vi "Initialize.vi"(8 "error in (no error)":errorcluster, 11 "Camera_Prime95B in":refnum<class "Camera_Prime95B.lvclass">) -> (0 "error out":errorcluster, 3 "Camera_Prime95B out":refnum<class "Camera_Prime95B.lvclass">)   [LabVIEW 2020, in "Camera_Prime95B.lvlib" / "Camera_Prime95B.lvclass"]
uses:
  Camera_Prime95B.lvclass
  E:/Development/DevHardSoftware/MicroscopyFramework/Model/Hardware Layer/Real Hardware/Camera_Prime95B/Camera_Prime95B/Dependencies/PVCamNET.dll
  Dependencies/PVCamNET.dll
  Hardware Abstraction Layer/Component/Camera/Camera/Camera.lvclass
  Hardware Abstraction Layer/Component/Device/Device/DeviceStatus.ctl
  Hardware Abstraction Layer/Component/Device/Device/Device.lvlib
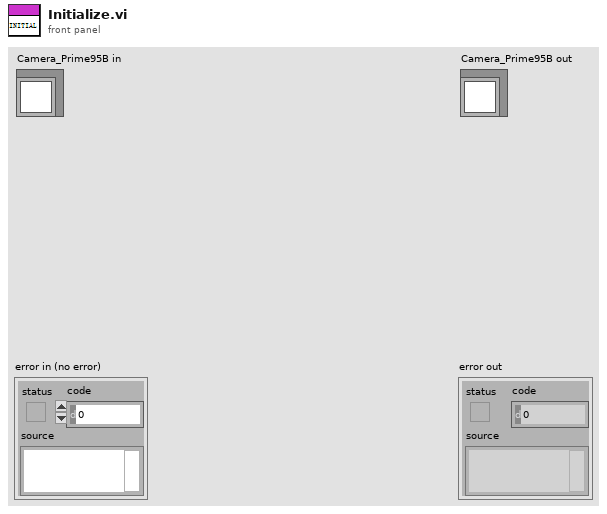
[diagram p1: front panel]
types:
  T1 = typedef "Device.lvlib/DeviceStatus.ctl" = i32
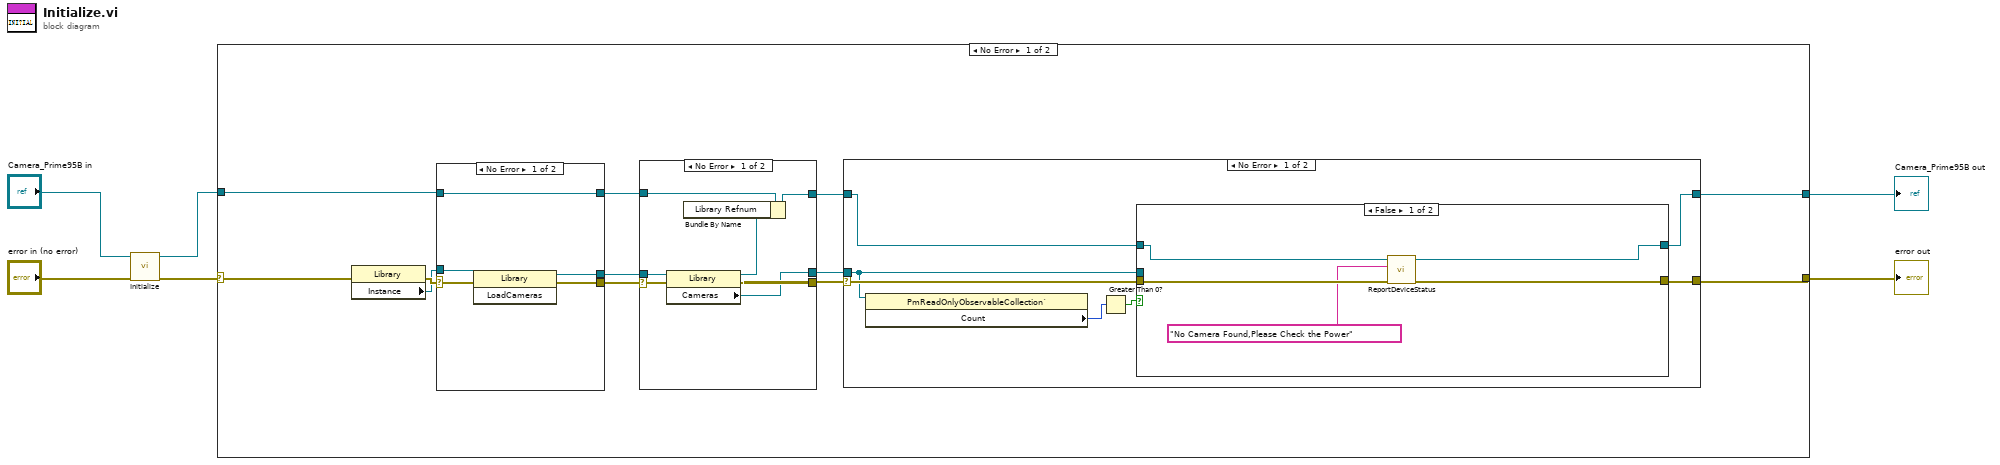
[diagram p0: block diagram]
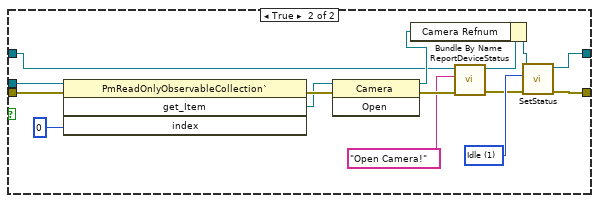
[diagram p2: hidden frame]
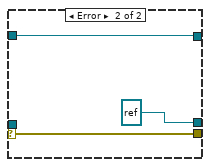
[diagram p4: hidden frame]
diagram:
  n1 = call-parent "Initialize.vi"("error in (no error)"="error in (no error)", "Camera in"="Camera_Prime95B in") -> ("error out"=w2:errorcluster, "Camera out"=w1:refnum<class "Camera_Prime95B.lvclass">)  [unwired: 8 in]
  n2 = case shown="No Error" w2 {
    selector: w2 -> [w12 w67]
    tunnel: [w8 w67] -> w5
    tunnel: w1 -> [w11 w66]
    tunnel: [w7 w66] -> w6
    frame No Error {
      n3 = property class="Library"(error in=w12) -> (error out=w18:errorcluster, "Instance"=w15:refnum<k24>)  [unwired: 1 in, 1 out]
      n4 = case shown="No Error" w18 {
        selector: w18 -> [w60 w65]
        tunnel: [w61 w65] -> w16
        tunnel: [w62 w64] -> w17
        tunnel: w15 -> [w59 w64]
        tunnel: w11 -> [w58 w63]
        tunnel: [w58 w63] -> w10
        frame No Error {
          n5 = invoke class="Library" method="LoadCameras"(reference=w59, error in=w60) -> (reference out=w62:refnum<k24>, error out=w61:errorcluster)  [unwired: 1 in, 1 out]
        }
        frame Error {
        }
      }
      n6 = case shown="No Error" w16 {
        selector: w16 -> [w54 w57]
        tunnel: [w52 w57] -> w13
        tunnel: w17 -> [w53 _]
        tunnel: [w51 refnum<k24> refnum ("Cameras")] -> w14
        tunnel: w10 -> [w50 w55]
        tunnel: [w49 w55] -> w9
        frame No Error {
          n7 = property class="Library"(reference=w53, error in=w54) -> (reference out=w48:refnum<k24>, error out=w52:errorcluster, "Cameras"=w51:refnum<k24>)
          n8 = Bundle By Name(cluster=w50, "Library Refnum"=w48) -> (w49:refnum<class "Camera_Prime95B.lvclass">)
        }
        frame Error {
        }
      }
      n9 = case shown="No Error" w13 {
        selector: w13 -> [w25 w47]
        tunnel: w14 -> [w21 _]
        tunnel: [w24 w47] -> w8
        tunnel: w9 -> [w20 w46]
        tunnel: [w19 w46] -> w7
        frame No Error {
          n10 = property class="PmReadOnlyObservableCollection`"(reference=w21) -> ("Count"=w22:i32)  [unwired: 1 in, 2 out]
          n11 = Greater Than 0?(x=w22) -> (x > 0?=w23:bool)
          n12 = case shown="False" w23 {
            tunnel: w25 -> [w30 w44]
            tunnel: [w29 w39] -> w24
            tunnel: w21 -> [_ w43]
            tunnel: w20 -> [w28 w33]
            tunnel: [w27 w38] -> w19
            frame False {
              n13 = call-dynamic "ReportDeviceStatus.vi"("error in (no error)"=w30, "Status"="No Camera Found,Please Check the Power", "Device in"=w28) -> ("error out"=w29:errorcluster, "Device out"=w27:refnum<class "Camera_Prime95B.lvclass">)  [unwired: 7 in]
            }
            frame True {
              w37 = T1 1 items=["Offline", "Idle", "Busy"] ("Status")
              n14 = invoke class="PmReadOnlyObservableCollection`" method="get_Item"(reference=w43, error in=w44, "index"=0) -> (error out=w42:errorcluster, "get_Item"=w40:refnum<k24>)  [unwired: 1 in, 2 out]
              n15 = invoke class="Camera" method="Open"(reference=w40, error in=w42) -> (reference out=w35:refnum<k24>, error out=w41:errorcluster)  [unwired: 1 in, 1 out]
              n16 = call-dynamic "ReportDeviceStatus.vi"("error in (no error)"=w41, "Status"="Open Camera!", "Device in"=w33) -> ("error out"=w34:errorcluster, "Device out"=w32:refnum<class "Camera_Prime95B.lvclass">)  [unwired: 7 in]
              n17 = Bundle By Name(cluster=w32, "Camera Refnum"=w35) -> (w36:refnum<class "Camera_Prime95B.lvclass">)
              n18 = call-dynamic "SetStatus.vi"("error in (no error)"=w34, "Status"=w37, "Device in"=w36) -> ("error out"=w39:errorcluster, "Device out"=w38:refnum<class "Camera_Prime95B.lvclass">)  [unwired: 7 in]
            }
          }
        }
        frame Error {
        }
      }
    }
    frame Error {
    }
  }
  "error out" <- w5
  "Camera_Prime95B out" <- w6
